vi "simulate hybrid DNA and WLC fit.vi"() -> ()   [LabVIEW 2014]
uses:
  <vilib>/gmath/NumericalOptimization/Nonlinear Curve Fit LM formula string.vi
  <vilib>/gmath/NI_Gmath.lvlib
panel:
  in  "Enum":enum16{"WLC", "modified WLC"}(ring)
  out "best fit parameters for eWLC 2":dbl[](array[numeric])
  in  "initial parameters for eWLC (Lc,Lp,K)":dbl[](array[numeric])=[1000.0, 1200.0]
  out "best fit parameters for eWLC":dbl[](array[numeric])
  out "best fit parameters for WLC":dbl[](array[numeric])
  in  "initial parameters for eWLC (Lc,K)":dbl[](array[numeric])=[1000.0, 1200.0]
  in  "initial parameters for WLC (Lp,Lc)":dbl[](array[numeric])=[45.0, 1800.0]
  in  "ssDNA Length (nt)":dbl
  in  "dsDNA Length (bp)":dbl
  out "expected contour length for ssDNA (nm) 2":dbl
  out "expected contour length for dsDNA (nm)":dbl
  in  "Tab Control":enum32{"Page 3", "Page 1"}(tab)
  out "Raw-XY Graph 2":cluster{dbl[], dbl[]}(graph)
  out "Fit-XY Graph":cluster{dbl[], "best nonlinear fit":dbl[]}[](graph)
  out "Force Array (pN)":dbl[](array[numeric])
  in  "End Force (pN)":dbl
  in  "dF (pN)":dbl
  in  "Start Force (pN)":dbl
  # "Lp=0.37 nm and Lc=0.28 nm for PEG"
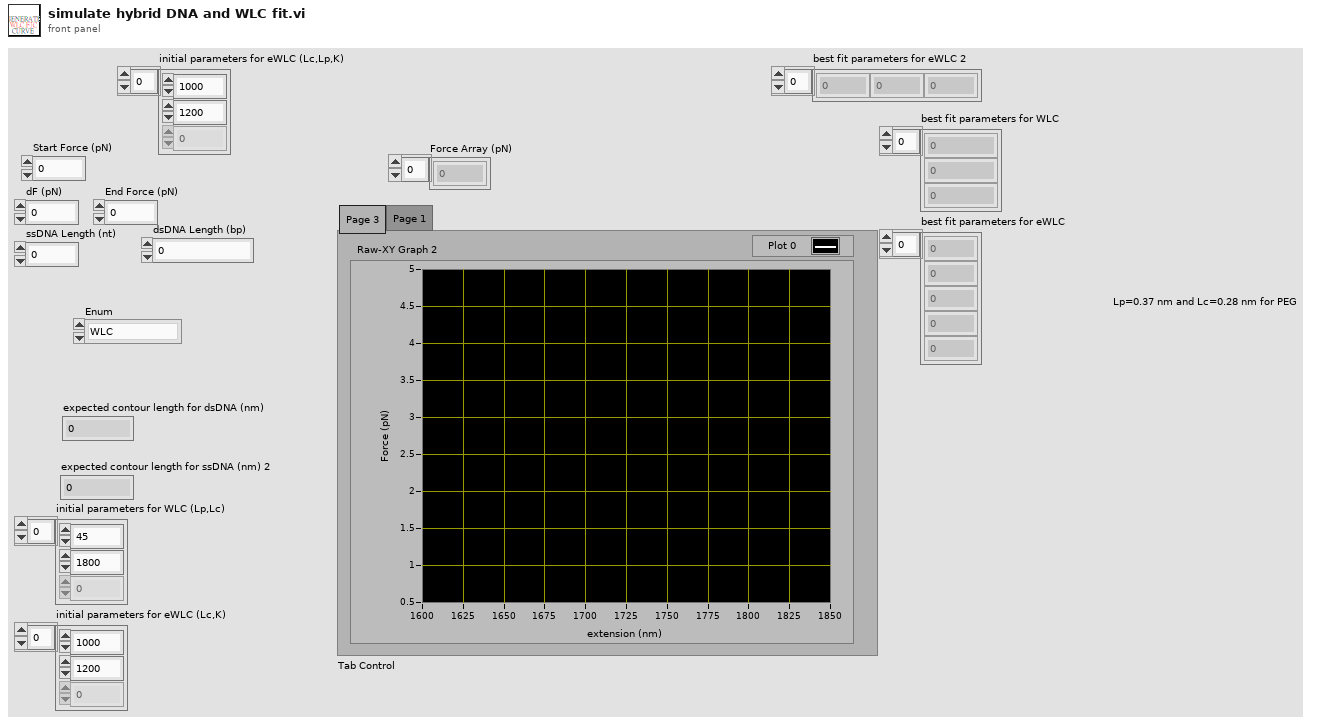
[diagram p1: front panel]
types:
  T1 = cluster{"model":string, "Parameters":string[], "x":string}
  T2 = cluster{"best nonlinear fit for eWLC":dbl[], "best nonlinear fit":dbl[]}
  T3 = cluster{"best nonlinear fit for eWLC":dbl[], "best nonlinear fit":dbl[]}[]
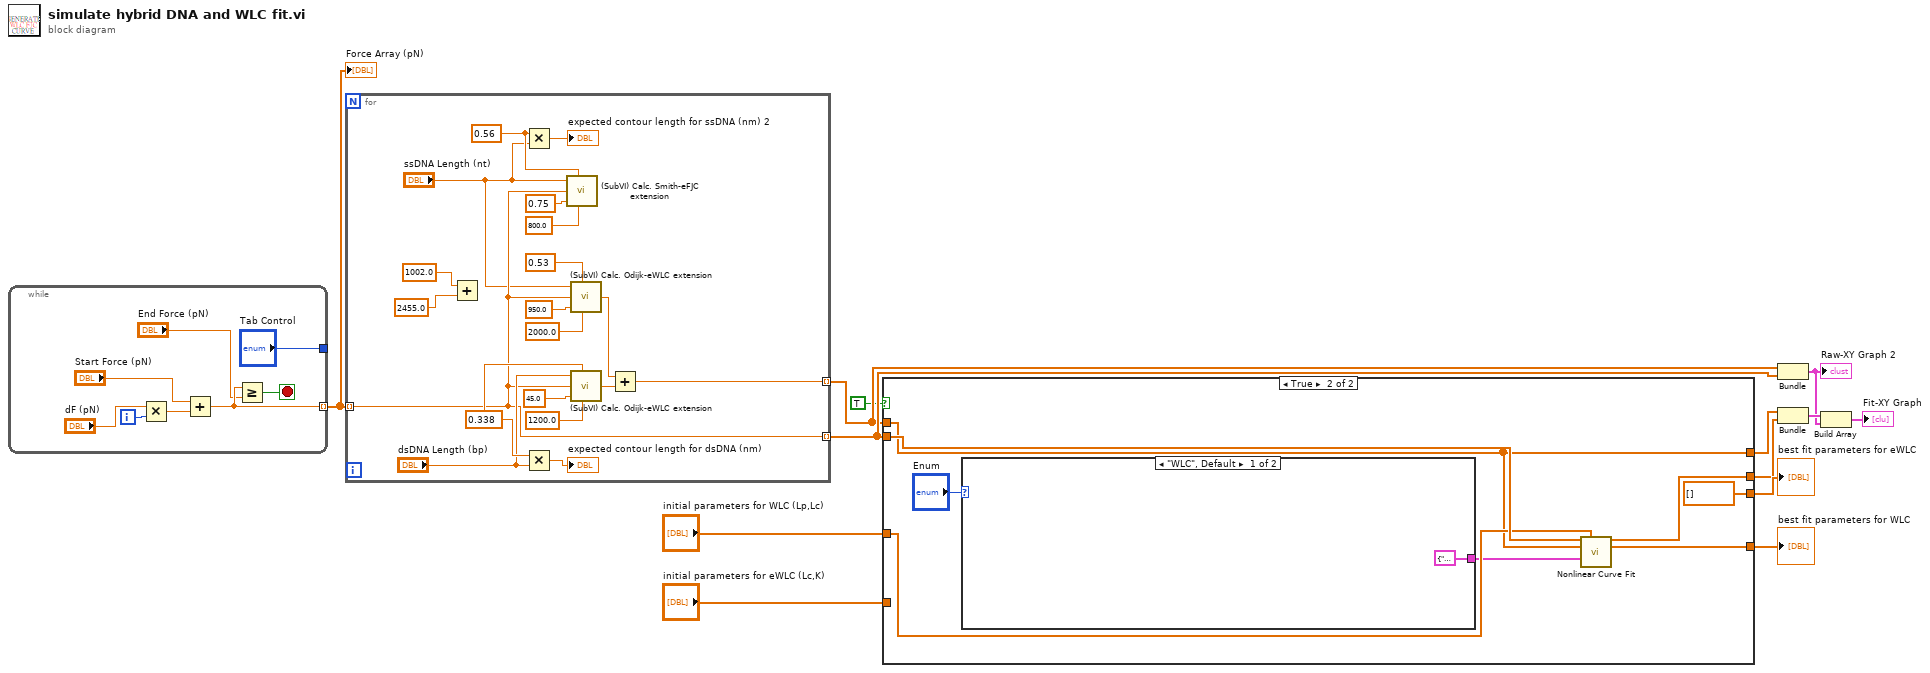
[diagram p0: block diagram]
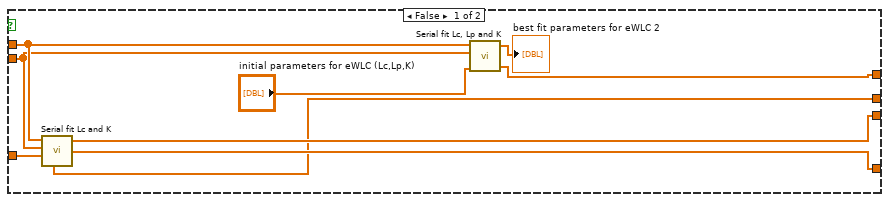
[diagram p2: hidden frame]
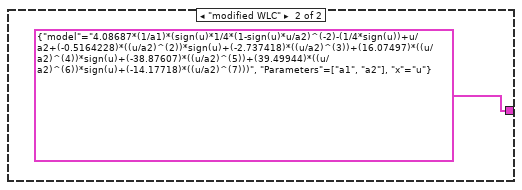
[diagram p3: hidden frame]
diagram:
  n1 = while {
    tunnel: [w17] -> w13 mode=indexing
    tunnel: ["Tab Control"] -> _
    i -> [w20]
    stop <- w15 stop-if-true
    n2 = Multiply(x="dF (pN)", y=w20) -> (x*y=w19:dbl)
    n3 = Add(x="Start Force (pN)", y=w19) -> (x+y=w17:dbl)
    n4 = Greater Or Equal?(x=w17, y="End Force (pN)") -> (x >= y?=w15:bool)
  }
  "Force Array (pN)" <- w13
  n5 = for {
    tunnel: w13 -> [w27] mode=indexing
    tunnel: [w40] -> w11 mode=indexing
    tunnel: [w27] -> w12 mode=indexing
    w39 = 0.338 ("nm/bp")
    w37 = 0.56 ("nm/nt")
    n6 = Add(x=1002.0 ("dsDNA Length (bp)"), y=2455.0 ("dsDNA Length (bp)")) -> ()  [unwired: 1 out]
    n7 = Multiply(x=w37, y="ssDNA Length (nt)") -> (x*y=→"expected contour length for ssDNA (nm) 2":dbl)
    n8 = Multiply(x=w39, y="dsDNA Length (bp)") -> (x*y=→"expected contour length for dsDNA (nm)":dbl)
    n9 = call "(SubVI) Calc. Smith-eFJC extension.vi"("ssDNA Length (nt)"="ssDNA Length (nt)", "nm/nt"=w37, "Force (pN)"=w27, "Persistence length (nm)"=0.75, "Elastic modulus (pN)"=800.0) -> ()  [unwired: 2 in, 1 out]
    n10 = call "(SubVI) Calc. Odijk-eWLC extension.vi"("dsDNA Length (bp)"="ssDNA Length (nt)", "nm/bp"=0.53, "Force (pN)"=w27, "Persistence length (nm)"=950.0, "Elastic modulus (pN)"=2000.0 ("Persistence length (nm)")) -> ("Extension (nm)"=w23:dbl)  [unwired: 2 in]
    n11 = call "(SubVI) Calc. Odijk-eWLC extension.vi"("dsDNA Length (bp)"="dsDNA Length (bp)", "nm/bp"=w39, "Force (pN)"=w27, "Persistence length (nm)"=45.0, "Elastic modulus (pN)"=1200.0) -> ("Extension (nm)"=w24:dbl)  [unwired: 2 in]
    n12 = Add(x=w23, y=w24) -> (x+y=w40:dbl)
  }
  n13 = case shown="True" TRUE {
    tunnel: w12 -> [w44 w57]
    tunnel: w11 -> [w45 w52]
    tunnel: [w41 w52] -> w2
    tunnel: "initial parameters for WLC (Lp,Lc)" -> [w49 w56]
    tunnel: "initial parameters for eWLC (Lc,K)" -> [_ _]
    tunnel: [w48 w55] -> w5
    tunnel: [w47 dbl[] [] ("best fit parameters for eWLC")] -> w4
    tunnel: [w46 w53] -> w1
    frame False {
      n14 = call "Serial fit Lc and K.vi"("Extension (nm)"=w45, "Force (pN)"=w44, "initial parameters for WLC (Lp,Lc)"=w49) -> ("Cut-Force (pN)"=w46:dbl[], "best fit parameters for eWLC (Lp,Lc,K)"=w47:dbl[], "best fit parameters for WLC"=w48:dbl[])  [unwired: 1 in, 2 out]
      n15 = call "Serial fit Lc, Lp and K.vi"("Extension (nm)"=w45, "Force (pN)"=w44, "initial parameters for eWLC (Lc,Lp,K)"="initial parameters for eWLC (Lc,Lp,K)") -> ("best fit parameters for eWLC"=→"best fit parameters for eWLC 2":dbl[], "best nonlinear fit for eWLC"=w41:dbl[])  [unwired: 3 in, 1 out]
    }
    frame True {
      n16 = case shown="\"WLC\", Default" "Enum" {
        tunnel: [T1 {"model"="4.08687*(1/a1)*(sign(u)*1/4*(1-sign(u)*u/a2)^(-2)-(1/4*sign(u))+u/a2)", "Parameters"=["a1", "a2"], "x"="u"} ("model description") T1 {"model"="4.08687*(1/a1)*(sign(u)*1/4*(1-sign(u)*u/a2)^(-2)-(1/4*sign(u))+u/a2+(-0.5164228)*((u/a2)^(2))*sign(u)+(-2.737418)*((u/a2)^(3))+(16.07497)*((u/a2)^(4))*sign(u)+(-38.87607)*((u/a2)^(5))+(39.49944)*((u/a2)^(6))*sign(u)+(-14.17718)*((u/a2)^(7)))", "Parameters"=["a1", "a2"], "x"="u"} ("model description")] -> w51
        frame "WLC", Default {
        }
        frame "modified WLC" {
        }
      }
      n17 = call-poly <vilib>:"Nonlinear Curve Fit.vi"("Y"=w57, "initial parameters"=w56, "X"=w52, "model description"=w51) -> ("best nonlinear fit"=w53:dbl[], "best fit parameters"=w55:dbl[])  [unwired: 3 in, 7 out]
    }
  }
  "best fit parameters for WLC" <- w5
  "best fit parameters for eWLC" <- w4
  n18 = Bundle(w11, w12) -> (w8:cluster{dbl[], dbl[]})  [unwired: 1 in]
  "Raw-XY Graph 2" <- w8
  n19 = Bundle("best nonlinear fit for eWLC"=w2, "best nonlinear fit"=w1) -> (w10:T2)  [unwired: 1 in]
  n20 = Build Array(w10, w8) -> (→"Fit-XY Graph":T3)
